vi "Pump Status FGV.vi"(7 "Write":bool, 8 "error in (no error)":errorcluster, 11 "Pump Status In":bool) -> (0 "error out":errorcluster, 3 "Pump Status Out":bool)   [LabVIEW 2018]
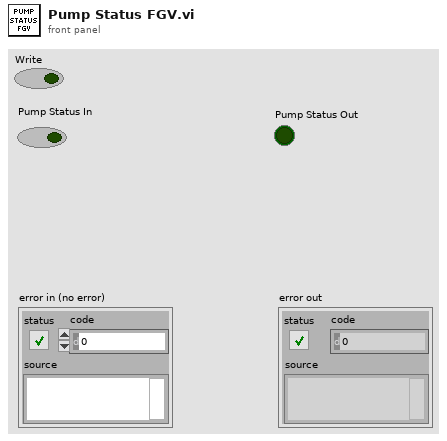
[diagram p1: front panel]
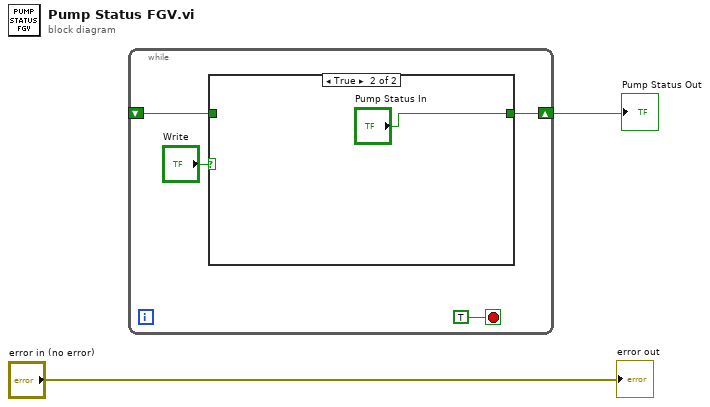
[diagram p0: block diagram]
diagram:
  n1 = while {
    shift-right: [w4] -> w1
    shift-left: _ -> [w3]
    stop <- TRUE stop-if-true
    n2 = case shown="True" "Write" {
      tunnel: [w7 "Pump Status In"] -> w4
      tunnel: w3 -> [w7 _]
      frame False {
      }
      frame True {
      }
    }
  }
  "Pump Status Out" <- w1
  "error out" <- "error in (no error)"
